vi "DAQallmethods.vi"(8 "error in":errorcluster, 9 "Index":dbl format="%#_13g", 10 "Parameters":T2, 11 "fromINIT":refnum<class "RADEBase.lvclass">) -> (0 "error out":errorcluster, 1 "Data Pack":T1, 3 "toExit":refnum<class "RADEBase.lvclass">)   [LabVIEW 2014]
uses:
  <userlib>/_RADE/RIO/RADEBase/classes/RADEBase/RADEBase.lvclass
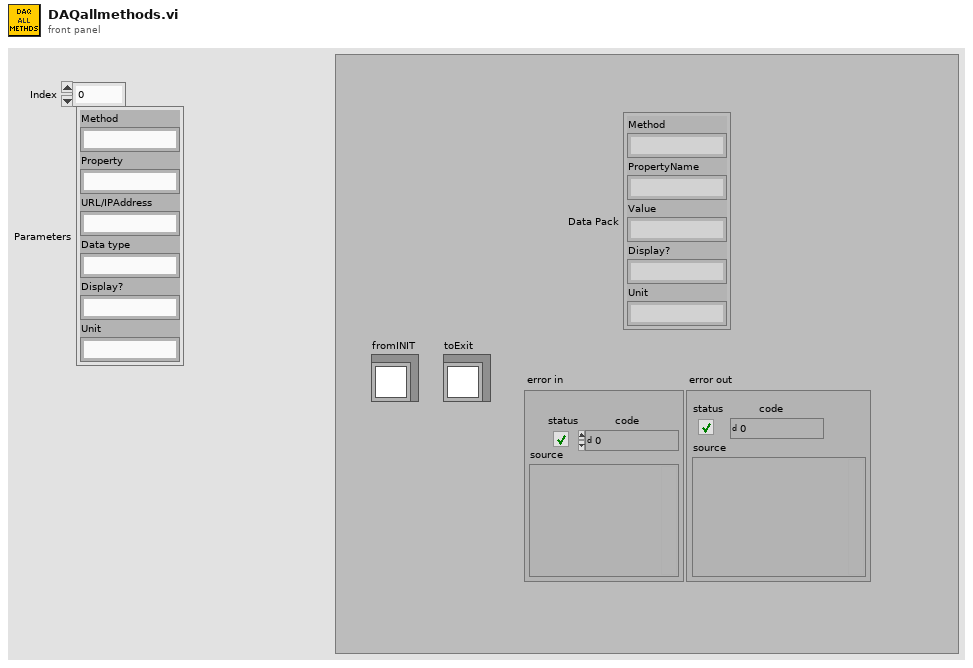
[diagram p1: front panel]
types:
  T1 = cluster{"Method":string, "PropertyName":string, "Value":string, "Display?":string, "Unit":string}
  T2 = cluster{"Method":string, "Property":string, "URL/IPAddress":string, "Data type":string, "Display?":string, "Unit":string}
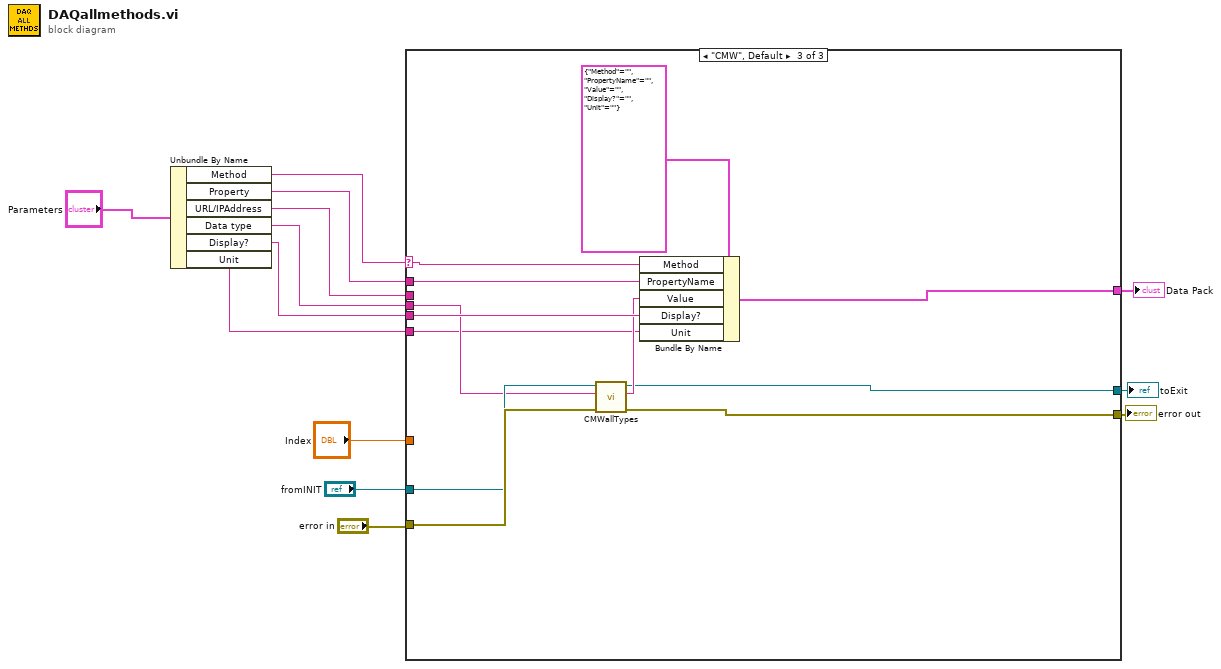
[diagram p0: block diagram]
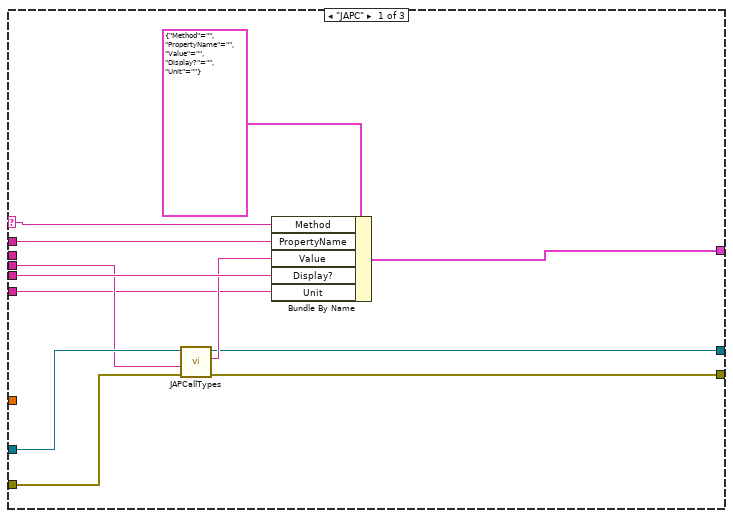
[diagram p2: hidden frame]
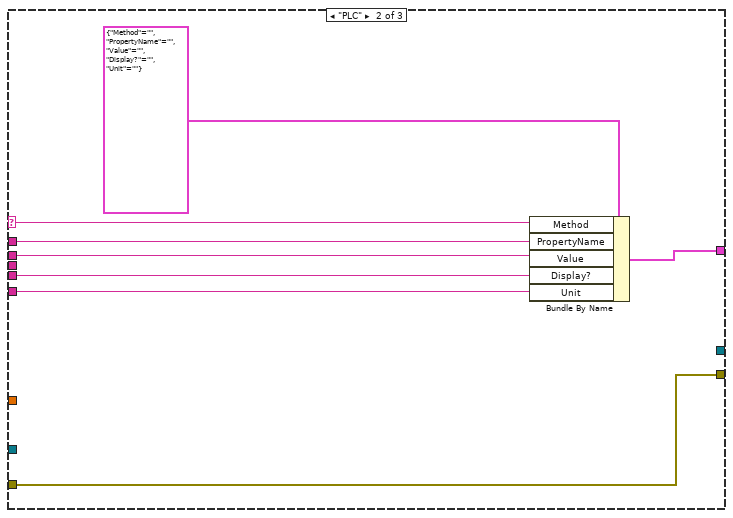
[diagram p3: hidden frame]
diagram:
  n1 = Unbundle By Name("Parameters") -> ("Method"=w12:string, "Property"=w11:string, "URL/IPAddress"=w10:string, "Data type"=w9:string, "Display?"=w8:string, "Unit"=w1:string)
  n2 = case shown="\"CMW\", Default" w12 {
    selector: w12 -> [w19 w29 w41]
    tunnel: "error in" -> [w25 w28 w45]
    tunnel: [w24 w28 w44] -> w13
    tunnel: w10 -> [_ w27 _]
    tunnel: w9 -> [w17 _ w37]
    tunnel: w11 -> [w20 w30 w40]
    tunnel: w8 -> [w23 w31 w42]
    tunnel: [w21 w32 w39] -> w2
    tunnel: "fromINIT" -> [w18 _ w38]
    tunnel: [w15 _ w35] -> w6
    tunnel: "Index" -> [_ _ _]
    tunnel: w1 -> [w14 w26 w34]
    frame "JAPC" {
      n3 = call "JAPCallTypes.vi"("error in (no error)"=w25, "Data Type"=w17, "JAPCinit"=w18) -> ("error out"=w24:errorcluster, "JAPCout"=w16:string, "JAPCexit"=w15:refnum<class "RADEBase.lvclass">)  [unwired: 6 in]
      n4 = Bundle By Name(cluster=T1 {"Method"="", "PropertyName"="", "Value"="", "Display?"="", "Unit"=""} ("input cluster"), "Method"=w19, "PropertyName"=w20, "Value"=w16, "Display?"=w23, "Unit"=w14) -> (w21:T1)
    }
    frame "PLC" {
      n5 = Bundle By Name(cluster=T1 {"Method"="", "PropertyName"="", "Value"="", "Display?"="", "Unit"=""} ("input cluster"), "Method"=w29, "PropertyName"=w30, "Value"=w27, "Display?"=w31, "Unit"=w26) -> (w32:T1)
    }
    frame "CMW", Default {
      n6 = call "CMWallTypes.vi"("error in"=w45, "Data Type"=w37, "CMWin"=w38) -> ("error out"=w44:errorcluster, "CMW"=w36:string, "CMWout"=w35:refnum<class "RADEBase.lvclass">)  [unwired: 6 in]
      n7 = Bundle By Name(cluster=T1 {"Method"="", "PropertyName"="", "Value"="", "Display?"="", "Unit"=""} ("input cluster"), "Method"=w41, "PropertyName"=w40, "Value"=w36, "Display?"=w42, "Unit"=w34) -> (w39:T1)
    }
  }
  "error out" <- w13
  "toExit" <- w6
  "Data Pack" <- w2
